vi "Perform_Meas_Setup.vi"(2 "Simulate/Run":T1, 3 "Traverse line":T2 {"Row Duration (mins)" format="%#.1f"; "Row No" min=0; "Trace Gas Concentration (%)" min=0.0 format="%#.2f"; "Emission Rate (l/min)" format="%#.2f"; "Tunnel Speed" format="%#.2f"; "Start X" format="%#.2f"; "Start Y" format="%#.2f"; "Start Z" format="%#.2f"; "End X" format="%#.2f"; "End Y" format="%#.2f"; "End Z" format="%#.2f"; "Averaging time (min)" min=0.0 format="%#.2f"}) -> (0 "Continue?":bool)   [LabVIEW 2010]
uses:
  Traverse_cluster.ctl
  Spacing.ctl
  Controls/Multi_run_mode.ctl
  Controls/User_Specific_mode.ctl
  File/Setup_Filetype.ctl
  Controls/Save_Data.ctl
  Controls/Setup.ctl
panel:
  # "X           Y            Z"
  # "Start"
  # "End"
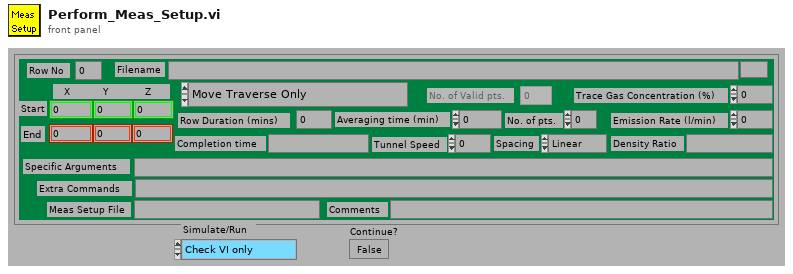
[diagram p1: front panel]
types:
  T1 = typedef "User_Specific_mode.ctl" = enum16{"Check VI only", "Run VI"}
  T2 = typedef "Traverse_cluster.ctl" = cluster{"Start X":dbl, "Start Y":dbl, "Start Z":dbl, "End X":dbl, "End Y":dbl, "End Z":dbl, "No. of pts.":i32, "Spacing":T3, "Filename":path, "Tunnel Speed":dbl, "Averaging time (min)":dbl, "Extra Commands":string, "Specific Arguments":string, "Emission Rate (l/min)":dbl, "Trace Gas Concentration (%)":dbl, "Density Ratio":string, "Comments":string, "Row No":i32, "Row Type Selector":T4, "Completion time":string, "Row Duration (mins)":dbl, "No. of Valid pts.":i32, "Meas Setup File":string}
  T3 = typedef "Spacing.ctl" = enum16{"Linear", "Log", "Gauss", "Specified", "N/A"}
  T4 = typedef "Multi_run_mode.ctl" = enum16{"Move Traverse Only", "Set Tunnel Speed Only", "Set Source Only", "Set Measurement Conditions", "Single Measurement", "Vertical Profile", "Lateral Profile", "Longitudinal Profile", "Explore Volume", "Multi-Axis Profile", "Auto Calibrate", "Meas Fast FID Bkgnd", "Check Beam Power", "Scanning Valve Measurement", "Run VI Named:", "Set ADAM Ch", "Wait (minutes)", "Send Message", "Synchronize With:", "Fall Back to this Row", "Turn Off Row Repeating", "Blank Row"}
  T5 = typedef "Setup_Filetype.ctl" = enum16{"Measurement Setups", "Calibration Setups", "General", "Results File Plotter Setups", "Speed Calib Tweaks"}
  T6 = typedef "Save_Data.ctl" = enum16{"Save No Data", "Save Data"}
  T7 = typedef "Setup.ctl" = enum16{"Run Program", "Show Setup", "Save Current Setup", "Setup Front Panel"}
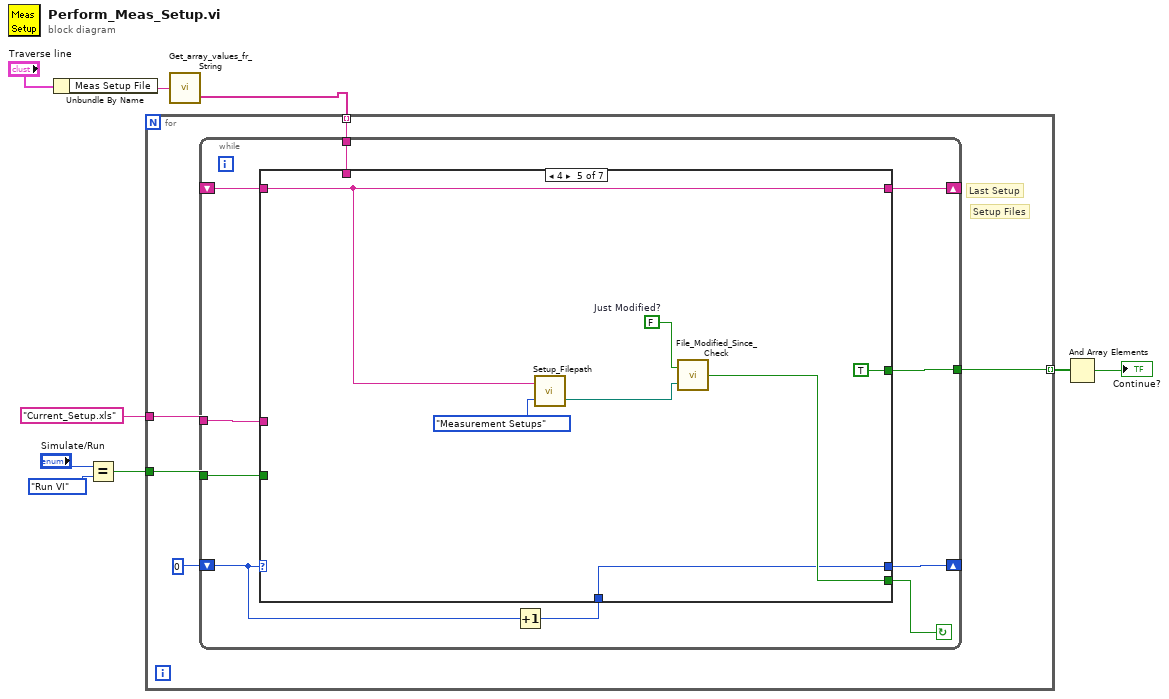
[diagram p0: block diagram]
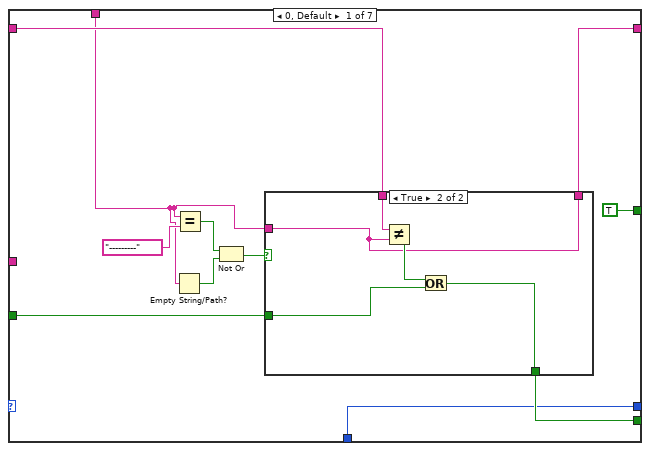
[diagram p2: hidden frame]
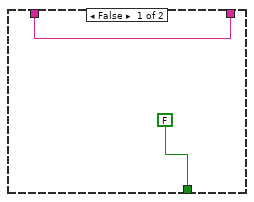
[diagram p3: hidden frame]
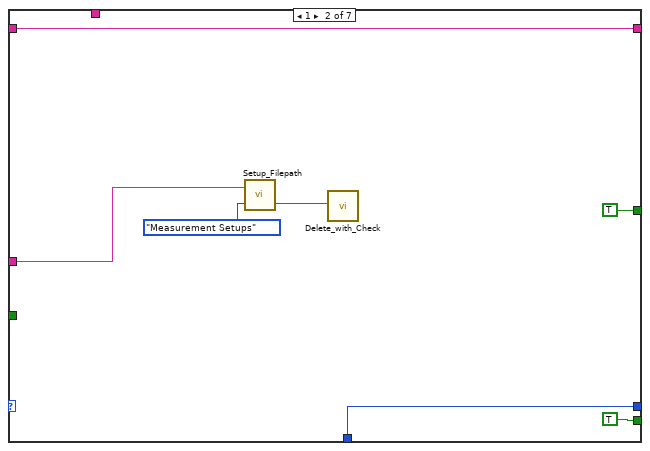
[diagram p4: hidden frame]
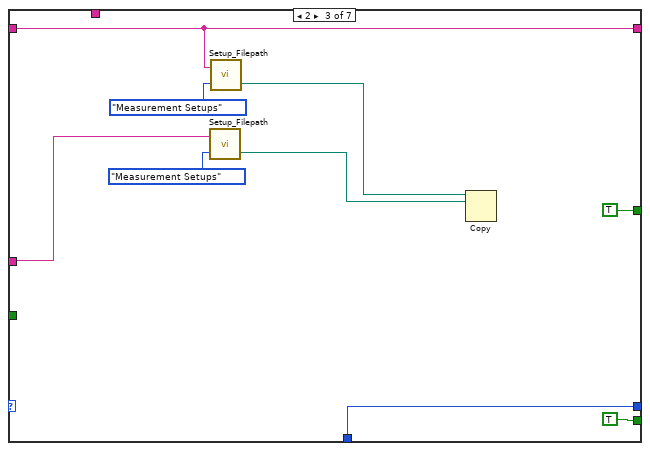
[diagram p5: hidden frame]
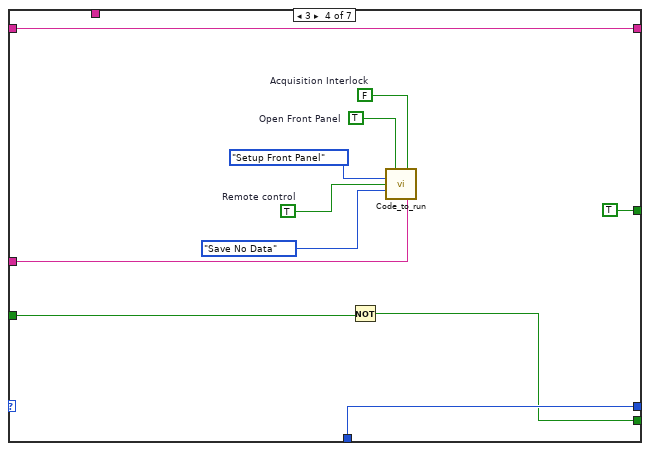
[diagram p6: hidden frame]
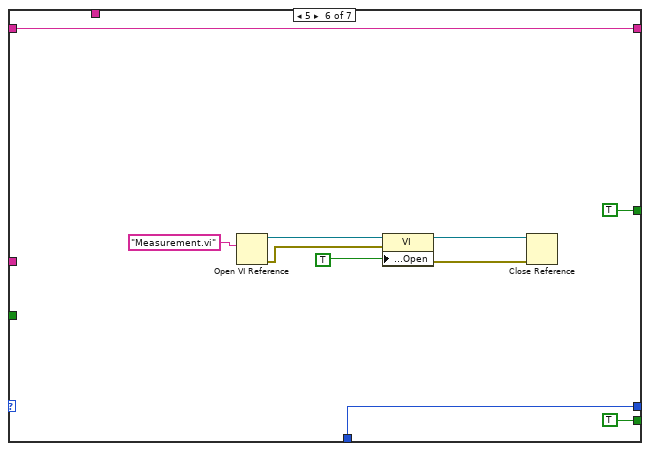
[diagram p7: hidden frame]
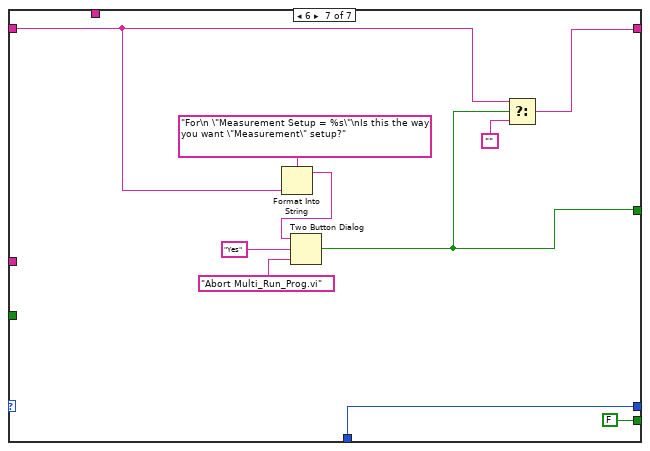
[diagram p8: hidden frame]
diagram:
  n1 = Unbundle By Name("Traverse line") -> ("Meas Setup File"=w4:string)
  n2 = Equal?(x="Simulate/Run", y=User_Specific_mode."Run VI" ("Simulate/Run")) -> (x = y?=w6:bool)
  n3 = call "Get_array_values_fr_String.vi"("String Value"=w4) -> ("String array"=w3:string[])  [unwired: 1 out]
  n4 = for {
    tunnel: "Current_Setup.xls" ("name or relative path") -> [w13]
    tunnel: w6 -> [w12]
    tunnel: w3 -> [w11] mode=indexing
    tunnel: [w10] -> w2 mode=indexing
    # "Last Setup"
    # "Setup Files"
    n5 = while {
      tunnel: w12 -> [w16]
      tunnel: w13 -> [w17]
      shift-left: _ -> [w19]
      shift-right: [w18] -> _
      tunnel: [w20] -> w10
      shift-left: 0 -> [w23]
      shift-right: [w21] -> _
      tunnel: w11 -> [w15]
      stop <- w24 continue-if-true
      n6 = Increment(x=w23) -> (x+1=w22:i32)
      n7 = case shown="4" w23 {
        tunnel: [w32 TRUE ("T button?") TRUE ("T button?") w61 w76 TRUE FALSE] -> w24
        tunnel: w22 -> [w30 w46 w56 w63 w75 w86 w96]
        tunnel: [w30 w46 w56 w63 w75 w86 w96] -> w21
        tunnel: [TRUE ("T button?") TRUE ("T button?") TRUE ("T button?") TRUE ("T button?") TRUE ("T button?") TRUE ("T button?") w90] -> w20
        tunnel: w19 -> [w34 w48 w53 w65 w71 w85 w88]
        tunnel: [w33 w48 w53 w65 w71 w85 w89] -> w18
        tunnel: w17 -> [_ w44 w51 w64 _ _ _]
        tunnel: w16 -> [w31 _ _ w62 _ _ _]
        tunnel: w15 -> [w25 _ _ _ _ _ _]
        frame 0, Default {
          n8 = Empty String/Path?(string/path=w25) -> (empty?=w27:bool)
          n9 = Equal?(x=w25, y="---------" ("f")) -> (x = y?=w28:bool)
          n10 = Not Or(1:w27, 2:w28) -> (0:w26:bool)
          n11 = case shown="True" w26 {
            tunnel: [w37 w39] -> w33
            tunnel: w25 -> [_ w39]
            tunnel: w34 -> [w37 w42]
            tunnel: [FALSE w40] -> w32
            tunnel: w31 -> [_ w38]
            frame False {
            }
            frame True {
              n12 = Not Equal?(x=w42, y=w39) -> (x != y?=w41:bool)
              n13 = Or(x=w41, y=w38) -> (x .or. y?=w40:bool)
            }
          }
        }
        frame 1 {
          n14 = call "Setup_Filepath.vi"("Setup File Type"=Setup_Filetype."Measurement Setups", "Filename in"=w44) -> ("Filename Out"=w43:path)  [unwired: 1 out]
          n15 = call "Delete_with_Check.vi"("FilePath"=w43) -> ()  [unwired: 1 out]
        }
        frame 2 {
          n16 = call "Setup_Filepath.vi"("Setup File Type"=Setup_Filetype."Measurement Setups", "Filename in"=w51) -> ("Filename Out"=w50:path)  [unwired: 1 out]
          n17 = call "Setup_Filepath.vi"("Setup File Type"=Setup_Filetype."Measurement Setups", "Filename in"=w53) -> ("Filename Out"=w52:path)  [unwired: 1 out]
          n18 = Copy(10:w50, 11:w52) -> ()  [unwired: 1 in, 5 out]
        }
        frame 3 {
          w66 = FALSE  # Acquisition Interlock
          w68 = TRUE  # Remote control
          w69 = TRUE  # Open Front Panel
          n19 = Not(x=w62) -> (.not. x?=w61:bool)
          n20 = call "Code_to_run.vi"("Open Front Panel"=w69, "Acquisition Interlock"=w66, "setup"=Setup."Setup Front Panel", "Remote control"=w68, "File"=Save_Data."Save No Data", "Setup filename"=w64) -> ()  [unwired: 4 in, 6 out]
        }
        frame 4 {
          w73 = FALSE  # Just Modified?
          n21 = call "Setup_Filepath.vi"("Setup File Type"=Setup_Filetype."Measurement Setups", "Filename in"=w71) -> ("Filename Out"=w70:path)  [unwired: 1 out]
          n22 = call "File_Modified_Since_Check.vi"("Pathname"=w70, "Just Modified?"=w73) -> ("Modified?"=w76:bool)
        }
        frame 5 {
          n23 = Open VI Reference(vi path="Measurement.vi") -> (vi reference=w81:refnum<vi>, error out=w82:errorcluster)  [unwired: 1 in, 4 out]
          n24 = property class="VI"(reference=w81, error in=w82, "Front Panel Window:Open"=TRUE) -> (reference out=w79:refnum<vi>, error out=w78:errorcluster)
          n25 = Close Reference(reference=w79, error in (no error)=w78) -> ()  [unwired: 1 out]
        }
        frame 6 {
          n26 = Format Into String(format string="For\n \"Measurement Setup = %s\"\nIs this the way you want \"Measurement\" setup?" ("message"), w88) -> (resulting string=w95:string)  [unwired: 2 in, 1 out]
          n27 = Two Button Dialog(message=w95, 1:"Abort Multi_Run_Prog.vi" ("F button name (\"Cancel\")"), 2:"Yes" ("T button name (\"OK\")")) -> (T button?=w90:bool)
          n28 = Select(t=w88, s=w90, f="") -> (s? t:f=w89:string)
        }
      }
    }
  }
  n29 = And Array Elements(Boolean array=w2) -> (logical AND=→"Continue?":bool)
